vi "Knob.vi"(0 "Freqin":dbl=1000.0 format="%_7g", 2 "Knob":i8(knob)=1 scale=1.0..20.0, 3 "Knob Step Size":i32(ring)=3 items=["1KHz", "10KHz", "100KHz", "1MHz", "10MHz", "100MHz", "1GHz"]) -> (8 "Freqout":dbl format="%_7g")   [LabVIEW 2017]
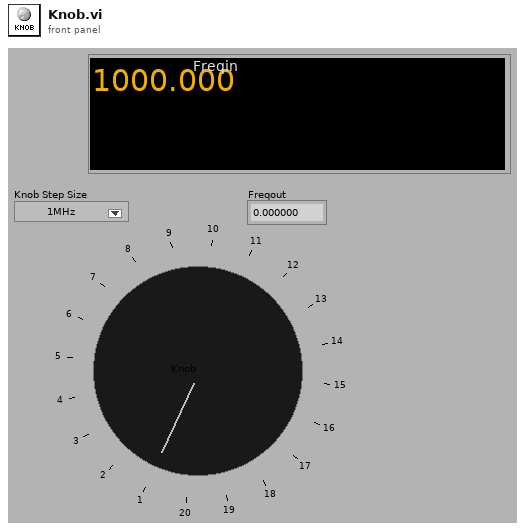
[diagram p1: front panel]
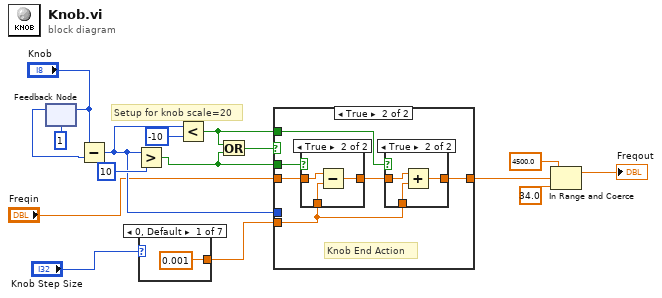
[diagram p0: block diagram]
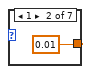
[diagram p2: hidden frame]
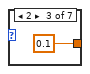
[diagram p3: hidden frame]
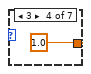
[diagram p4: hidden frame]
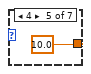
[diagram p5: hidden frame]
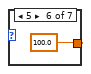
[diagram p6: hidden frame]
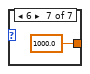
[diagram p7: hidden frame]
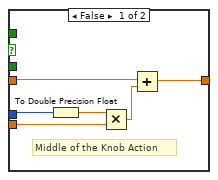
[diagram p8: hidden frame]
diagram:
  # "Setup for knob scale=20"
  n1 = feedback-in #1("Knob") -> ()
  n2 = feedback #1(i8 1 ("Knob")) -> (w6:i8)
  n3 = Subtract(x="Knob", y=w6) -> (x-y=w4:i8)
  n4 = Greater?(x=w4, y=10) -> (0:w13:bool)
  n5 = case shown="0, Default" "Knob Step Size" {
    tunnel: [0.001 0.01 0.1 1.0 10.0 100.0 1000.0] -> w10
    frame 0, Default {
    }
    frame 1 {
    }
    frame 2 {
    }
    frame 3 {
    }
    frame 4 {
    }
    frame 5 {
    }
    frame 6 {
    }
  }
  n6 = Less?(x=w4, y=-10) -> (x < y?=w12:bool)
  n7 = Or(x=w12, y=w13) -> (x .or. y?=w14:bool)
  n8 = case shown="True" w14 {
    tunnel: w13 -> [_ w35]
    tunnel: "Freqin" -> [w28 w34]
    tunnel: w12 -> [_ w32]
    tunnel: [w29 w31] -> w2
    tunnel: w10 -> [w27 w30]
    tunnel: w4 -> [w24 _]
    frame False {
      # "Middle of the Knob Action"
      n9 = To Double Precision Float(number=w24) -> (double precision float=w25:dbl)
      n10 = Multiply(x=w25, y=w27) -> (x*y=w26:dbl)
      n11 = Add(x=w28, y=w26) -> (x+y=w29:dbl)
    }
    frame True {
      # "Knob End Action"
      n12 = case shown="True" w35 {
        tunnel: w34 -> [w40 w42]
        tunnel: [w40 w43] -> w33
        tunnel: w30 -> [_ w41]
        frame False {
        }
        frame True {
          n13 = Subtract(x=w42, y=w41) -> (x-y=w43:dbl)
        }
      }
      n14 = case shown="True" w32 {
        tunnel: w33 -> [w36 w38]
        tunnel: [w36 w39] -> w31
        tunnel: w30 -> [_ w37]
        frame False {
        }
        frame True {
          n15 = Add(x=w38, y=w37) -> (x+y=w39:dbl)
        }
      }
    }
  }
  n16 = In Range and Coerce(upper limit=4500.0, x=w2, lower limit=34.0) -> (coerced(x)=→"Freqout":dbl)  [unwired: 1 out]
